vi "Position_Checker.vi"(7 "Car Position Slider":u8(slide) scale=0.0..4.0, 8 "error in (no error)":errorcluster, 11 "Current Station":T1) -> (0 "error out":errorcluster, 3 "Out of Position":bool)   [LabVIEW 2020]
doc: "This VI looks at wash stage and determines if the car is in the right position"
uses:
  Controls/Queue_Control.ctl
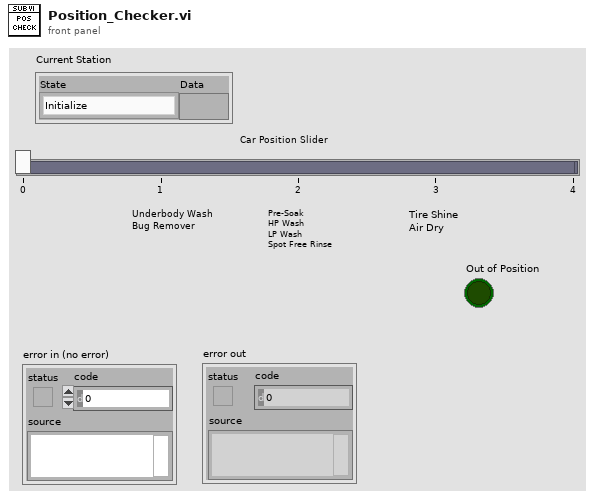
[diagram p1: front panel]
types:
  T1 = typedef "Queue_Control.ctl" = cluster{"State":enum16{"Initialize", "Start", "Next Station", "Under Body Wash", "Bug Remover", "Pre-soak", "High Pressure Wash", "Low Pressure Wash", "Spot Free Rinse", "Tire Shine Foam", "Air Dry", "Exit", "Check Position", "Out of Position", "Stop"}, "Data":variant}
  T2 = enum16{"Initialize", "Start", "Next Station", "Under Body Wash", "Bug Remover", "Pre-soak", "High Pressure Wash", "Low Pressure Wash", "Spot Free Rinse", "Tire Shine Foam", "Air Dry", "Exit", "Check Position", "Out of Position", "Stop"}
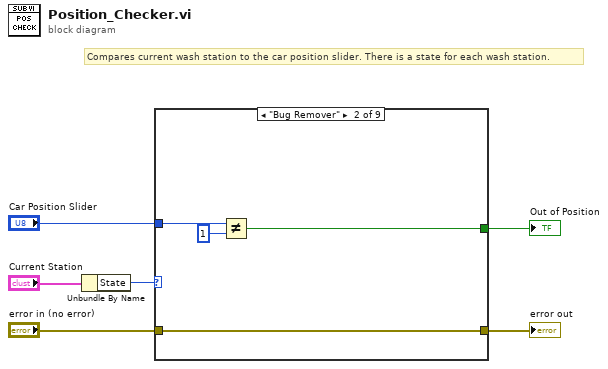
[diagram p0: block diagram]
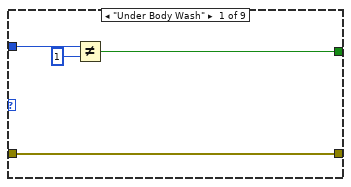
[diagram p2: hidden frame]
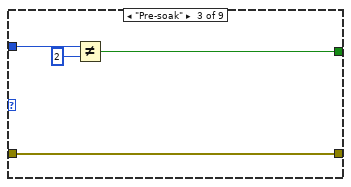
[diagram p3: hidden frame]
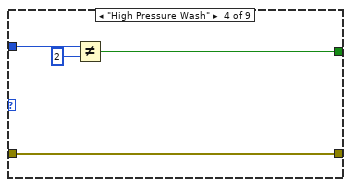
[diagram p4: hidden frame]
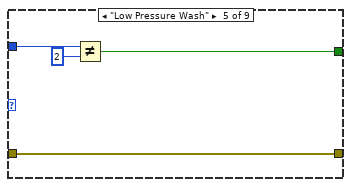
[diagram p5: hidden frame]
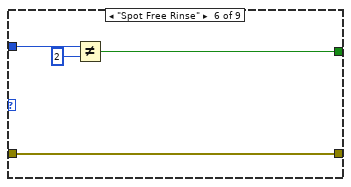
[diagram p6: hidden frame]
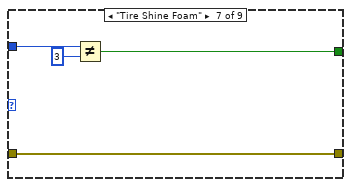
[diagram p7: hidden frame]
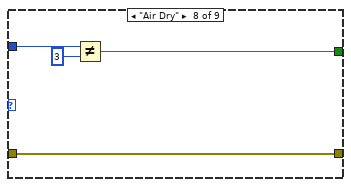
[diagram p8: hidden frame]
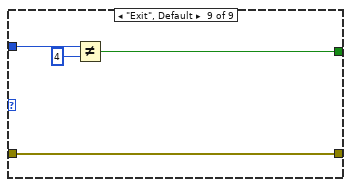
[diagram p9: hidden frame]
diagram:
  # "Compares current wash station to the car position slider. There is a state for each wash station."
  n1 = Unbundle By Name("Current Station") -> ("State"=w1:T2)
  n2 = case shown="\"Bug Remover\"" w1 {
    tunnel: "Car Position Slider" -> [w10 w14 w18 w22 w26 w30 w34 w38 w42]
    tunnel: [w8 w12 w16 w20 w24 w28 w32 w36 w40] -> w6
    tunnel: "error in (no error)" -> [w7 w11 w15 w19 w23 w27 w31 w35 w39]
    tunnel: [w7 w11 w15 w19 w23 w27 w31 w35 w39] -> w4
    frame "Under Body Wash" {
      n3 = Not Equal?(x=w10, y=u8 1) -> (x != y?=w8:bool)
    }
    frame "Bug Remover" {
      n4 = Not Equal?(x=w14, y=u8 1) -> (x != y?=w12:bool)
    }
    frame "Pre-soak" {
      n5 = Not Equal?(x=w18, y=u8 2) -> (x != y?=w16:bool)
    }
    frame "High Pressure Wash" {
      n6 = Not Equal?(x=w22, y=u8 2) -> (x != y?=w20:bool)
    }
    frame "Low Pressure Wash" {
      n7 = Not Equal?(x=w26, y=u8 2) -> (x != y?=w24:bool)
    }
    frame "Spot Free Rinse" {
      n8 = Not Equal?(x=w30, y=u8 2) -> (x != y?=w28:bool)
    }
    frame "Tire Shine Foam" {
      n9 = Not Equal?(x=w34, y=u8 3) -> (x != y?=w32:bool)
    }
    frame "Air Dry" {
      n10 = Not Equal?(x=w38, y=u8 3) -> (x != y?=w36:bool)
    }
    frame "Exit", Default {
      n11 = Not Equal?(x=w42, y=u8 4) -> (x != y?=w40:bool)
    }
  }
  "Out of Position" <- w6
  "error out" <- w4
